vi "channeldata_timestamp.vi"() -> ()   [LabVIEW 2019]
panel:
  out "Error Out":errorcluster
  in  "TDMS File":path=path "C:/Python/projects/nitdms/tests/tdms_files/channeldata_timestamp.tdms"
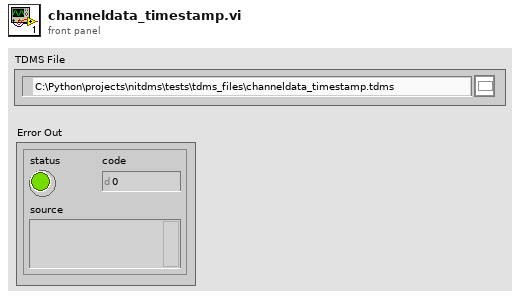
[diagram p1: front panel]
types:
  T1 = enum16{"open", "open or create", "create or replace", "create", "open (read-only)"}
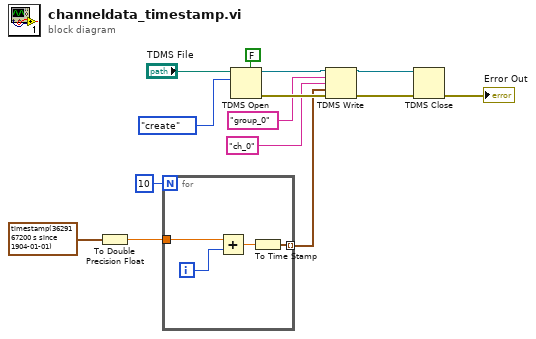
[diagram p0: block diagram]
diagram:
  n1 = To Double Precision Float(number=timestamp(3629167200 s since 1904-01-01)) -> (double precision float=w2:dbl)
  n2 = for {
    N: 10 -> [_]
    tunnel: w2 -> [w18]
    tunnel: [w15] -> w1 mode=indexing
    i -> [w17]
    n3 = Add(x=w18, y=w17) -> (x+y=w16:dbl)
    n4 = To Time Stamp(1:w16) -> (0:w15:timestamp)
  }
  n5 = TDMS Open(5:FALSE ("create index file? (T)"), 10:T1."create" ("operation (0:open)"), 11:"TDMS File") -> (0:w10:errorcluster, 3:w9:refnum<k34>)  [unwired: 4 in]
  n6 = TDMS Write(0:w9, 5:"group_0", 7:"ch_0", 9:w1, 11:w10) -> (4:w7:refnum<k34>, 15:w8:errorcluster)  [unwired: 1 in, 2 out]
  n7 = TDMS Close(8:w8, 11:w7) -> (0:→"Error Out":errorcluster)  [unwired: 1 out]
